vi "CDK_RW_Project_BuildInfo.vi"(7 "StorageAction":T2, 8 "ErrIn":errorcluster, 10 "BldInfoIn":T1[](array[typedef]), 11 "WizardIn":T3) -> (0 "ErrOut":errorcluster, 2 "BldInfoOut":T1[](array[typedef]), 3 "WizardOut":T3)   [LabVIEW 2020]
uses:
  <resource>/Framework/Providers/Builds/Installer/CDK_sTypeDef_StorageReadWrite.ctl
  <resource>/Framework/Providers/API/ItemRef.ctl
  <resource>/Framework/Providers/Builds/Installer/CDK_sTypeDef_BuildInfo.ctl
panel:
  in  "Template":T1
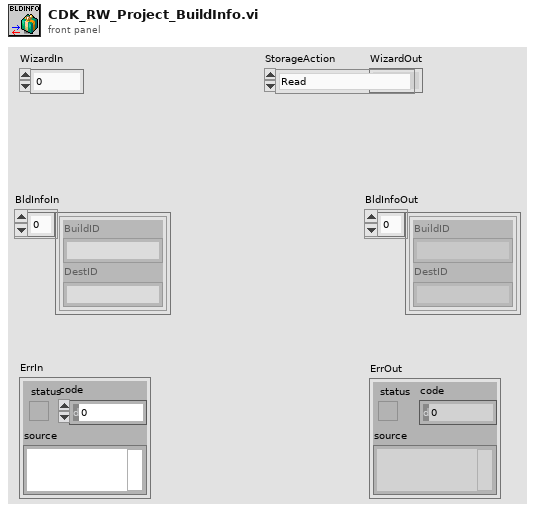
[diagram p1: front panel]
types:
  T1 = typedef "CDK_sTypeDef_BuildInfo.ctl" = cluster{"BuildID":string, "DestID":string}
  T2 = typedef "CDK_sTypeDef_StorageReadWrite.ctl" = enum16{"Read", "Write", "Empty", "readPrevious"}
  T3 = typedef "ItemRef.ctl" = u64
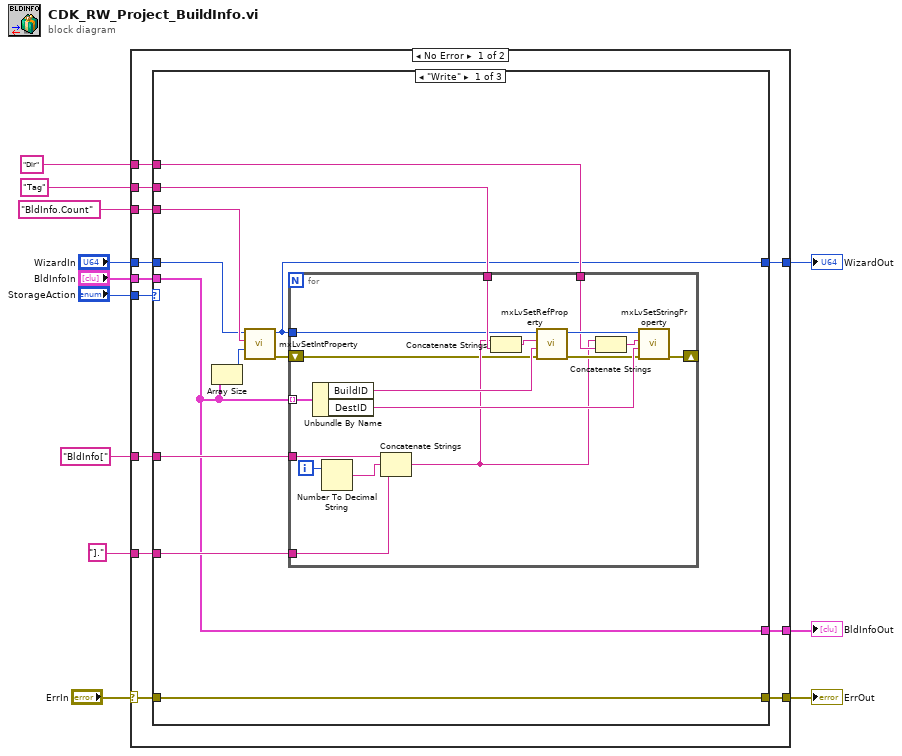
[diagram p0: block diagram]
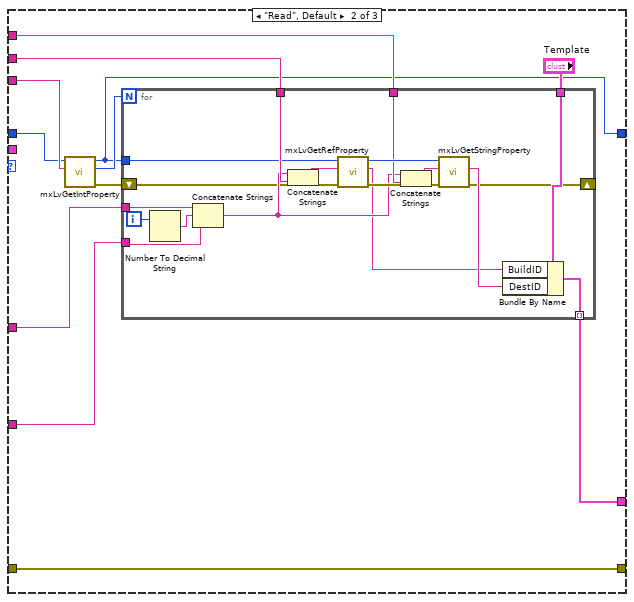
[diagram p2: hidden frame]
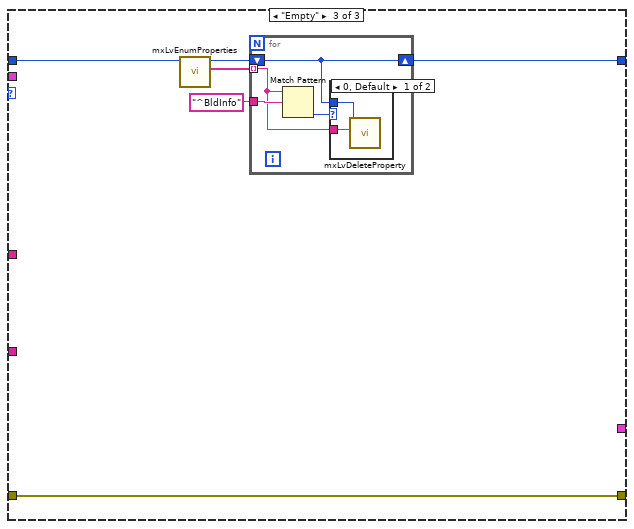
[diagram p3: hidden frame]
diagram:
  n1 = case shown="No Error" "ErrIn" {
    selector: "ErrIn" -> [w21 w97]
    tunnel: [w20 w97] -> w11
    tunnel: "StorageAction" -> [w24 _]
    tunnel: "WizardIn" -> [w23 w96]
    tunnel: "BldInfoIn" -> [w22 w95]
    tunnel: [w19 w96] -> w8
    tunnel: [w18 w95] -> w1
    tunnel: "BldInfo.Count" ("Tag") -> [w17 _]
    tunnel: "Tag" ("Tag") -> [w16 _]
    tunnel: "Dir" ("Tag") -> [w15 _]
    tunnel: "BldInfo[" -> [w14 _]
    tunnel: "]." -> [w13 _]
    frame No Error {
      n2 = case shown="\"Write\"" w24 {
        tunnel: w23 -> [w26 w54 w88]
        tunnel: w22 -> [w25 _ _]
        tunnel: w21 -> [w35 w64 w83]
        tunnel: [w35 w64 w83] -> w20
        tunnel: [w30 w55 w84] -> w19
        tunnel: [w25 w53 _] -> w18
        tunnel: w17 -> [w33 w62 _]
        tunnel: w16 -> [w32 w61 _]
        tunnel: w15 -> [w31 w60 _]
        tunnel: w14 -> [w28 w57 _]
        tunnel: w13 -> [w27 w56 _]
        frame "Write" {
          n3 = Array Size(array=w25) -> (size(s)=w34:i32)
          n4 = call <resource>:"mxLvSetIntProperty.vi"("Value (0)"=w34, "Tag"=w33, "Item"=w26) -> ("error out"=w29:errorcluster, "Item"=w30:T3)  [unwired: 2 in, 5 out]
          n5 = for {
            tunnel: w25 -> [w52] mode=indexing
            tunnel: w28 -> [w50]
            tunnel: w27 -> [w48]
            tunnel: w30 -> [w37]
            tunnel: w32 -> [w41]
            tunnel: w31 -> [w40]
            shift-right: [w36] -> _
            shift-left: w29 -> [w38]
            i -> [w51]
            n6 = Unbundle By Name(w52) -> ("BuildID"=w43:string, "DestID"=w44:string)
            n7 = Number To Decimal String(number=w51) -> (decimal integer string=w49:string)  [unwired: 1 out]
            n8 = Concatenate Strings(w50, w49, w48) -> (w39:string)
            n9 = Concatenate Strings(w39, w41) -> (w47:string)
            n10 = call <resource>:"mxLvSetRefProperty.vi"("error in"=w38, "Value (\"\")"=w43, "Tag"=w47, "Item"=w37) -> ("error out"=w42:errorcluster, "Item"=w45:T3)  [unwired: 1 in, 5 out]
            n11 = Concatenate Strings(w39, w40) -> (w46:string)
            n12 = call <resource>:"mxLvSetStringProperty.vi"("error in"=w42, "Value (\"\")"=w44, "Tag"=w46, "Item"=w45) -> ("error out"=w36:errorcluster)  [unwired: 1 in, 6 out]
          }
        }
        frame "Read", Default {
          n13 = call <resource>:"mxLvGetIntProperty.vi"("Tag"=w62, "Item"=w54) -> ("error out"=w58:errorcluster, "Value"=w63:i32, "Item"=w55:T3)  [unwired: 1 in, 6 out]
          n14 = for {
            N: w63 -> [_]
            tunnel: w57 -> [w81]
            tunnel: w56 -> [w79]
            tunnel: w55 -> [w67]
            tunnel: w61 -> [w70]
            tunnel: w60 -> [w71]
            tunnel: [w74] -> w53 mode=indexing
            tunnel: "Template" -> [w73]
            shift-right: [w66] -> _
            shift-left: w58 -> [w68]
            i -> [w82]
            n15 = Number To Decimal String(number=w82) -> (decimal integer string=w80:string)  [unwired: 1 out]
            n16 = Concatenate Strings(w81, w80, w79) -> (w69:string)
            n17 = Concatenate Strings(w69, w70) -> (w78:string)
            n18 = call <resource>:"mxLvGetRefProperty.vi"("Error In"=w68, "Tag"=w78, "Item"=w67) -> ("Error Out"=w72:errorcluster, "Value"=w65:string, "Item"=w76:T3)  [unwired: 6 out]
            n19 = Concatenate Strings(w69, w71) -> (w77:string)
            n20 = call <resource>:"mxLvGetStringProperty.vi"("Error In"=w72, "Tag"=w77, "Item"=w76) -> ("Error Out"=w66:errorcluster, "Value"=w75:string)  [unwired: 7 out]
            n21 = Bundle By Name(cluster=w73, "BuildID"=w65, "DestID"=w75) -> (w74:T1)
          }
        }
        frame "Empty" {
          n22 = call <resource>:"mxLvEnumProperties.vi"("Item"=w88) -> ("Property Tags"=w87:string[], "Item"=w86:T3)  [unwired: 1 in, 8 out]
          n23 = for {
            tunnel: w87 -> [w91] mode=indexing
            tunnel: "^BldInfo" -> [w92]
            shift-right: [w89] -> w84
            shift-left: w86 -> [w89]
            n24 = Match Pattern(string=w91, regular expression=w92) -> (offset past match=w90:i32)  [unwired: 4 out]
            n25 = case shown="0, Default" w90 {
              tunnel: w91 -> [w94 _]
              tunnel: w89 -> [w93 _]
              frame 0, Default {
                n26 = call <resource>:"mxLvDeleteProperty.vi"("Tag"=w94, "Item"=w93) -> ()  [unwired: 1 in, 9 out]
              }
              frame -1 {
              }
            }
          }
        }
      }
    }
    frame Error {
    }
  }
  "WizardOut" <- w8
  "ErrOut" <- w11
  "BldInfoOut" <- w1
